vi "Util_Trajectory_WriteFile_PathFinderConfig.vi"(9 "UTIL_PATHFINDER_CONFIG":T1 {"ActualMaxVelocity-inches per sec" format="%21.5f"; "WheelbaseDepth-inches" format="%21.5f"; "WheelbaseWidth-inches" format="%21.5f"; "TimeDelta-Seconds" format="%21.5f"; "MaxJerk--Inches per sec2" format="%21.5f"; "MaxAcceleration - inches per sec2" format="%21.5f"; "PathMaxVelocity - inches per sec" format="%21.5f"}, 11 "Byte Steam File In":refnum<file>) -> (0 "error out":errorcluster, 3 "Byte Steam File Out":refnum<file>)   [LabVIEW 2019, in "Trajectory_Library.lvlib"]
doc: "Internal routine to write the Pathfinder configuration to a file. This can be used on a PC or the RoboRIO.\n\nParameters:\n - ByteStreamIn - file stream\n - PathfinderConfig - cluster with configuration information.\n\nReturns:\n - ByteStreamOut - File stream.\n - Error out - returned error cluster\n\nReturns:\n - outTrajectory - Trajectory data structure\n - Error out - returned error cluster"
uses:
  Trajectory_Library.lvlib
  UTIL_PATHFINDER_CONFIG.ctl
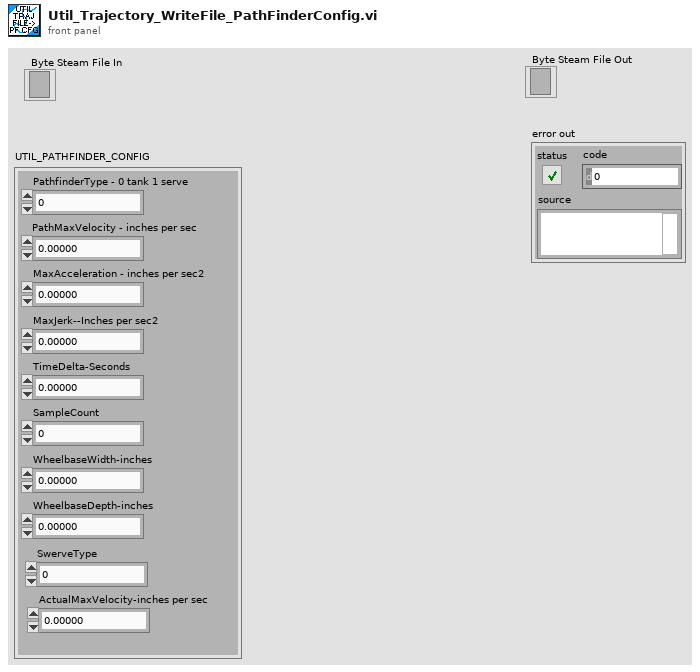
[diagram p1: front panel]
types:
  T1 = typedef "Trajectory_Library.lvlib/UTIL_PATHFINDER_CONFIG.ctl" = cluster{"PathfinderType - 0 tank 1 serve":i32, "PathMaxVelocity - inches per sec":dbl, "MaxAcceleration - inches per sec2":dbl, "MaxJerk--Inches per sec2":dbl, "TimeDelta-Seconds":dbl, "SampleCount":i32, "WheelbaseWidth-inches":dbl, "WheelbaseDepth-inches":dbl, "SwerveType":i32, "ActualMaxVelocity-inches per sec":dbl}
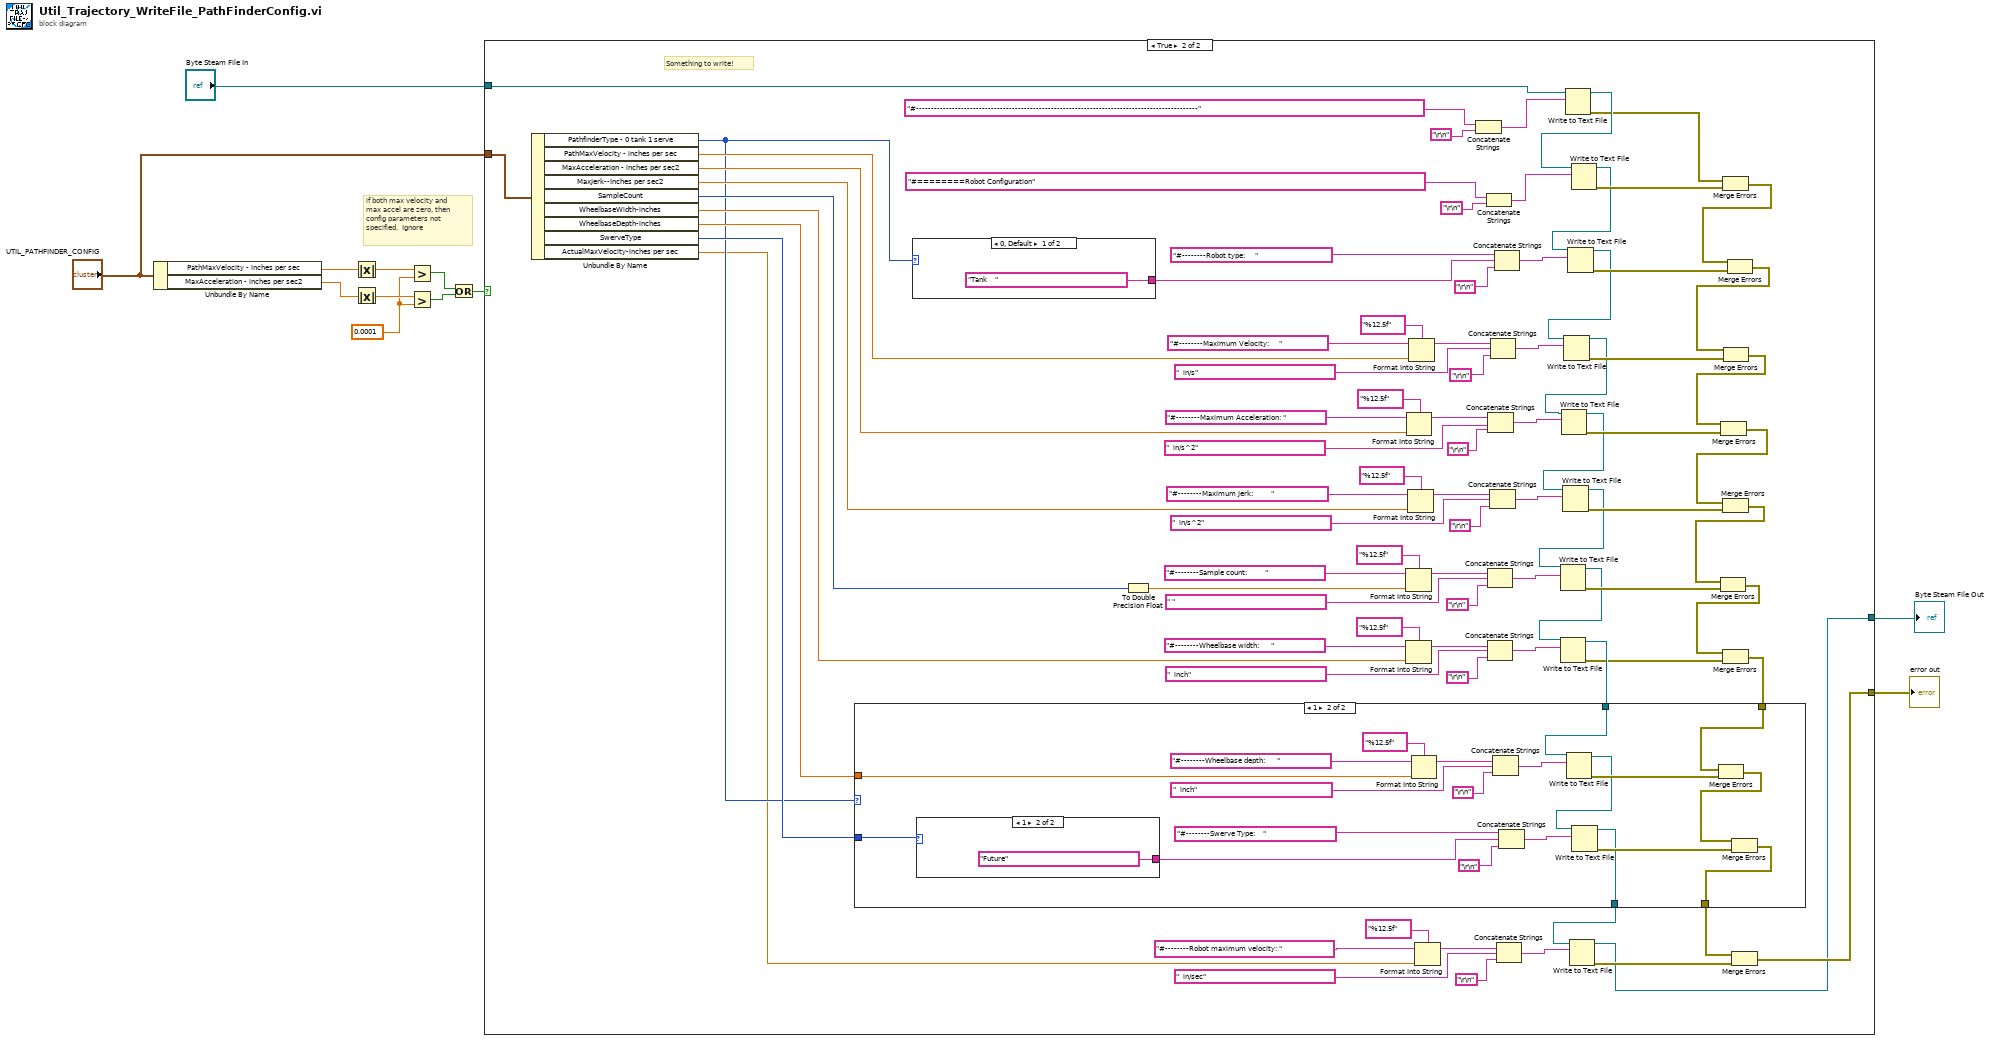
[diagram p0: block diagram]
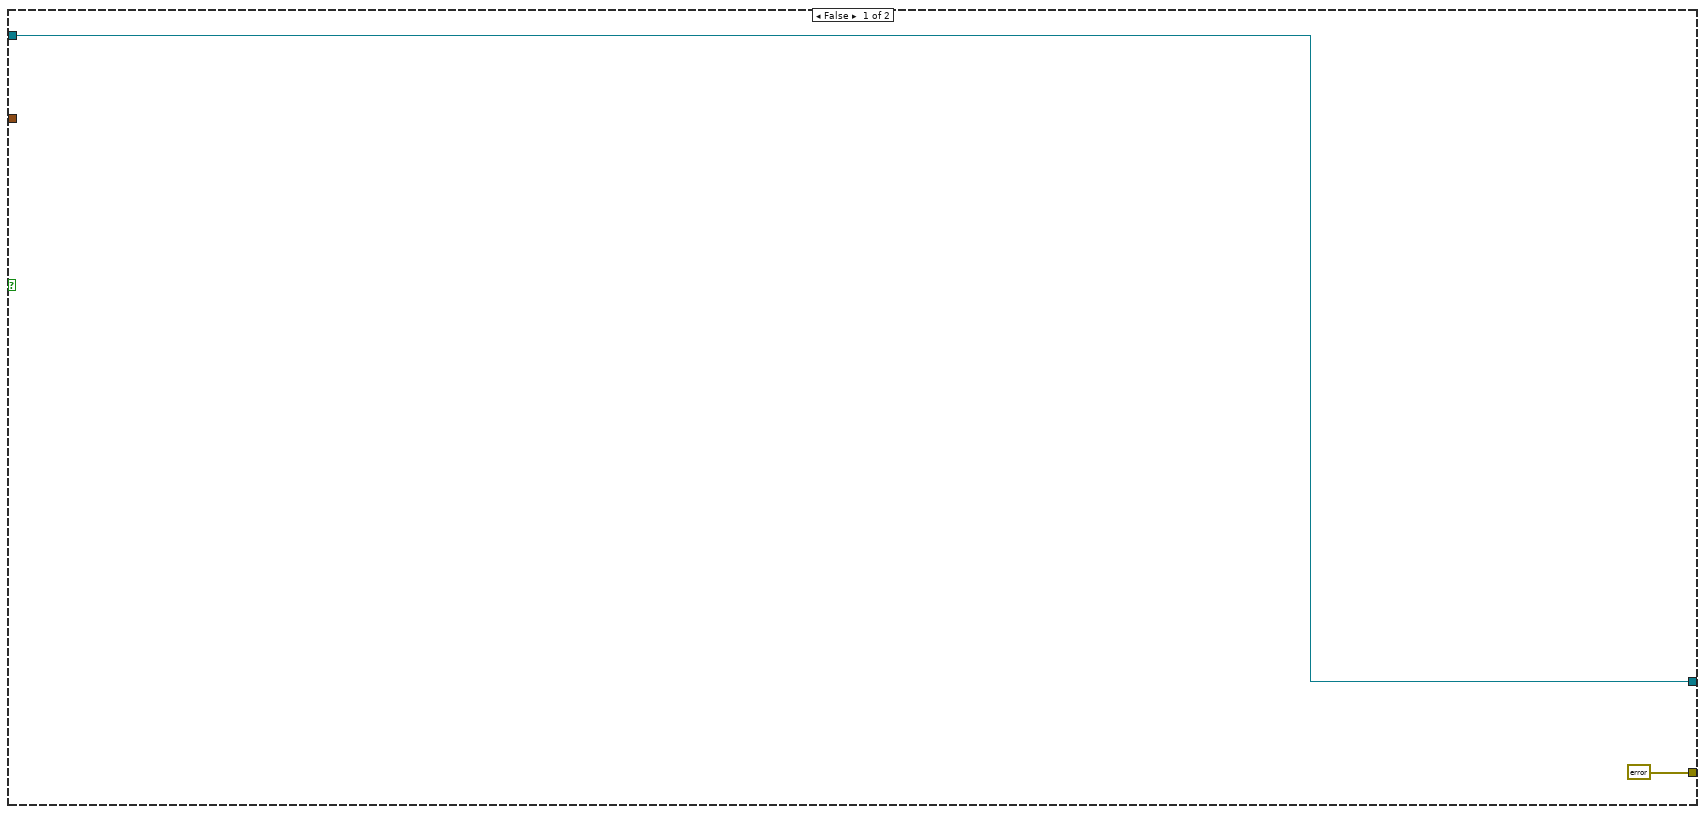
[diagram p2: hidden frame]
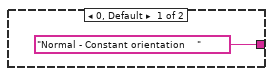
[diagram p4: hidden frame]
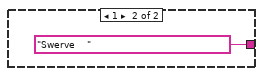
[diagram p5: hidden frame]
diagram:
  w5 = 0.0001
  # "if both max velocity and\nmax accel are zero, then\nconfig parameters not\nspecified.  Ignore"
  n1 = Unbundle By Name("UTIL_PATHFINDER_CONFIG") -> ("PathMaxVelocity - inches per sec"=w8:dbl, "MaxAcceleration - inches per sec2"=w9:dbl)
  n2 = Absolute Value(x=w8) -> (abs(x)=w7:dbl)
  n3 = Absolute Value(x=w9) -> (abs(x)=w6:dbl)
  n4 = Greater?(x=w7, y=w5) -> (0:w4:bool)
  n5 = Greater?(x=w6, y=w5) -> (0:w3:bool)
  n6 = Or(x=w4, y=w3) -> (x .or. y?=w2:bool)
  n7 = case shown="True" w2 {
    tunnel: [w14 w16] -> w12
    tunnel: "Byte Steam File In" -> [w14 w94]
    tunnel: [errorcluster {"status"=FALSE, "code"=0, "source"=""} ("error out") w17] -> w10
    tunnel: "UTIL_PATHFINDER_CONFIG" -> [_ w62]
    frame False {
    }
    frame True {
      # "Something to write!"
      n8 = Unbundle By Name(w62) -> ("PathfinderType - 0 tank 1 serve"=w27:i32, "PathMaxVelocity - inches per sec"=w53:dbl, "MaxAcceleration - inches per sec2"=w52:dbl, "MaxJerk--Inches per sec2"=w51:dbl, "SampleCount"=w49:i32, "WheelbaseWidth-inches"=w40:dbl, "WheelbaseDepth-inches"=w39:dbl, "SwerveType"=w28:i32, "ActualMaxVelocity-inches per sec"=w15:dbl)
      n9 = case shown="0, Default" w27 {
        tunnel: ["Tank    " ("string") "Swerve    " ("string")] -> w29
        frame 0, Default {
        }
        frame 1 {
        }
      }
      n10 = To Double Precision Float(number=w49) -> (double precision float=w50:dbl)
      n11 = Format Into String(format string="%12.5f", initial string="#--------Sample count:         " ("string"), w50) -> (resulting string=w71:string)  [unwired: 1 in, 1 out]
      n12 = Format Into String(format string="%12.5f", initial string="#--------Wheelbase width:      " ("string"), w40) -> (resulting string=w45:string)  [unwired: 1 in, 1 out]
      n13 = Format Into String(format string="%12.5f", initial string="#--------Maximum Acceleration: " ("string"), w52) -> (resulting string=w81:string)  [unwired: 1 in, 1 out]
      n14 = Format Into String(format string="%12.5f", initial string="#--------Maximum Jerk:         " ("string"), w51) -> (resulting string=w76:string)  [unwired: 1 in, 1 out]
      n15 = Format Into String(format string="%12.5f", initial string="#--------Maximum Velocity:     " ("string"), w53) -> (resulting string=w86:string)  [unwired: 1 in, 1 out]
      n16 = Format Into String(format string="%12.5f", initial string="#--------Robot maximum velocity: " ("string"), w15) -> (resulting string=w23:string)  [unwired: 1 in, 1 out]
      n17 = Concatenate Strings("#----------------------------------------------------------------------------------------------" ("string"), "\r\n") -> (w95:string)
      n18 = Concatenate Strings("#========Robot Configuration" ("string"), "\r\n") -> (w98:string)
      n19 = Concatenate Strings(w71, " " ("string"), "\r\n") -> (w73:string)
      n20 = Concatenate Strings(w45, "  inch" ("string"), "\r\n") -> (w46:string)
      n21 = Concatenate Strings(w81, "  in/s^2" ("string"), "\r\n") -> (w83:string)
      n22 = Concatenate Strings(w76, "  in/s^2" ("string"), "\r\n") -> (w78:string)
      n23 = Concatenate Strings(w86, "  in/s" ("string"), "\r\n") -> (w90:string)
      n24 = Concatenate Strings("#--------Robot type:     " ("string"), w29, "\r\n") -> (w37:string)
      n25 = Concatenate Strings(w23, "  in/sec" ("string"), "\r\n") -> (w24:string)
      n26 = Write to Text File(file (use dialog)=w94, text=w95) -> (refnum out=w93:refnum<file>, error out=w87:errorcluster)  [unwired: 2 in, 1 out]
      n27 = Write to Text File(file (use dialog)=w93, text=w98) -> (refnum out=w33:refnum<file>, error out=w89:errorcluster)  [unwired: 2 in, 1 out]
      n28 = Write to Text File(file (use dialog)=w33, text=w37) -> (refnum out=w32:refnum<file>, error out=w36:errorcluster)  [unwired: 2 in, 1 out]
      n29 = Write to Text File(file (use dialog)=w32, text=w90) -> (refnum out=w61:refnum<file>, error out=w88:errorcluster)  [unwired: 2 in, 1 out]
      n30 = Write to Text File(file (use dialog)=w61, text=w83) -> (refnum out=w60:refnum<file>, error out=w82:errorcluster)  [unwired: 2 in, 1 out]
      n31 = Write to Text File(file (use dialog)=w60, text=w78) -> (refnum out=w59:refnum<file>, error out=w77:errorcluster)  [unwired: 2 in, 1 out]
      n32 = Write to Text File(file (use dialog)=w59, text=w73) -> (refnum out=w42:refnum<file>, error out=w72:errorcluster)  [unwired: 2 in, 1 out]
      n33 = Write to Text File(file (use dialog)=w42, text=w46) -> (refnum out=w41:refnum<file>, error out=w38:errorcluster)  [unwired: 2 in, 1 out]
      n34 = Merge Errors(w87, w89) -> (w31:errorcluster)
      n35 = Merge Errors(w31, w36) -> (w30:errorcluster)
      n36 = Merge Errors(w30, w88) -> (w58:errorcluster)
      n37 = Merge Errors(w58, w82) -> (w57:errorcluster)
      n38 = Merge Errors(w57, w77) -> (w56:errorcluster)
      n39 = Merge Errors(w56, w72) -> (w55:errorcluster)
      n40 = Merge Errors(w55, w38) -> (w54:errorcluster)
      n41 = case shown="1" w27 {
        tunnel: w54 -> [w101 w122]
        tunnel: w41 -> [w102 w115]
        tunnel: w39 -> [_ w114]
        tunnel: w28 -> [_ w105]
        tunnel: [w102 w104] -> w19
        tunnel: [w101 w103] -> w18
        frame 0, Default {
        }
        frame 1 {
          n42 = case shown="1" w105 {
            tunnel: ["Normal - Constant orientation    " ("string") "Future" ("string")] -> w108
            frame 0, Default {
            }
            frame 1 {
            }
          }
          n43 = Format Into String(format string="%12.5f", initial string="#--------Wheelbase depth:      " ("string"), w114) -> (resulting string=w118:string)  [unwired: 1 in, 1 out]
          n44 = Concatenate Strings(w118, "  inch" ("string"), "\r\n") -> (w119:string)
          n45 = Concatenate Strings("#--------Swerve Type:    " ("string"), w108, "\r\n") -> (w112:string)
          n46 = Write to Text File(file (use dialog)=w115, text=w119) -> (refnum out=w106:refnum<file>, error out=w113:errorcluster)  [unwired: 2 in, 1 out]
          n47 = Write to Text File(file (use dialog)=w106, text=w112) -> (refnum out=w104:refnum<file>, error out=w111:errorcluster)  [unwired: 2 in, 1 out]
          n48 = Merge Errors(w122, w113) -> (w107:errorcluster)
          n49 = Merge Errors(w107, w111) -> (w103:errorcluster)
        }
      }
      n50 = Write to Text File(file (use dialog)=w19, text=w24) -> (refnum out=w16:refnum<file>, error out=w20:errorcluster)  [unwired: 2 in, 1 out]
      n51 = Merge Errors(w18, w20) -> (w17:errorcluster)
    }
  }
  "error out" <- w10
  "Byte Steam File Out" <- w12
